vi "Add to Channel.vi"(0 "reference fpga in":refnum<class "niUSRP Reference FPGA v1.lvclass">, 5 "collection builder in":refnum<class "Collection Builder.lvclass">) -> (4 "reference fpga out":refnum<class "niUSRP Reference FPGA v1.lvclass">)   [LabVIEW 2025, in "niUSRP Reference FPGA v1.lvclass"]
uses:
  niUSRP Reference FPGA v1.lvclass
  <instrlib>/_niInstr/Instruction Framework/v1/FPGA/Collection Builder/Collection Builder.lvclass
  niUSRP Reference FPGA v1.lvclass/niUSRP Reference FPGA v1.ctl
  <instrlib>/_niInstr/Instruction Framework/v1/FPGA/Top Level Bus/Register Configuration/Register Configuration.lvclass
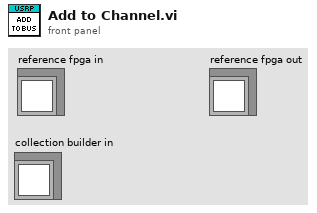
[diagram p1: front panel]
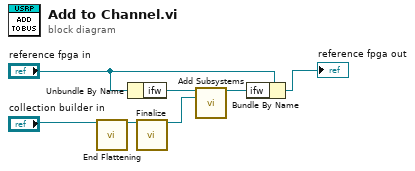
[diagram p0: block diagram]
diagram:
  n1 = call <instrlib>:"End Flattening.vi"("collection builder in"="collection builder in") -> ("collection builder out"=w2:refnum<class "Collection Builder.lvclass">)  [unwired: 14 in]
  n2 = Unbundle By Name("reference fpga in") -> ("ifw"=w4:refnum<class "Register Configuration.lvclass">)
  n3 = call <instrlib>:"Finalize.vi"("collection builder in"=w2) -> ("address space collection"=w1:refnum<class "Address Space Collection.lvclass">)  [unwired: 14 in]
  n4 = call-dynamic "Add Subsystems.vi"("register configuration in"=w4, "subsystems"=w1) -> ("register configuration out"=w5:refnum<class "Register Configuration.lvclass">)  [unwired: 13 in]
  n5 = Bundle By Name(cluster="reference fpga in", "ifw"=w5) -> (→"reference fpga out":refnum<class "niUSRP Reference FPGA v1.lvclass">)
